vi "Check Buffer Size (Base 2).vi"(5 "source vi name":string, 6 "bytes to move":u64 format="%d bytes", 7 "power of 2":i16, 8 "error in (no error)":errorcluster, 9 "offset (0)":u64 format="%d bytes", 10 "buffer count":u64 format="%d elements", 11 "Pointer in":refnum<class "Pointer.lvclass">) -> (0 "error out":errorcluster, 1 "offset":u64 format="%d bytes", 2 "buffer count":u64 format="%d elements", 3 "Pointer out":refnum<class "Pointer.lvclass">)   [LabVIEW 2017, in "Memory Manager.lvlib" / "Pointer.lvclass"]
uses:
  Pointer.lvclass
  Buffer Underflow.vi
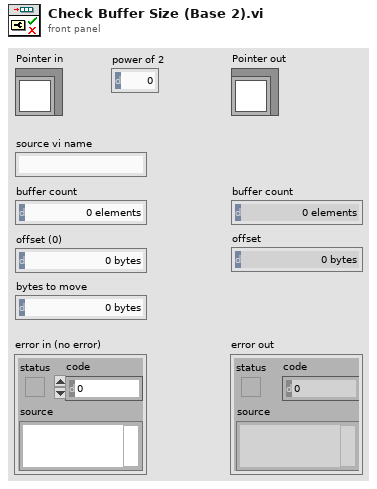
[diagram p1: front panel]
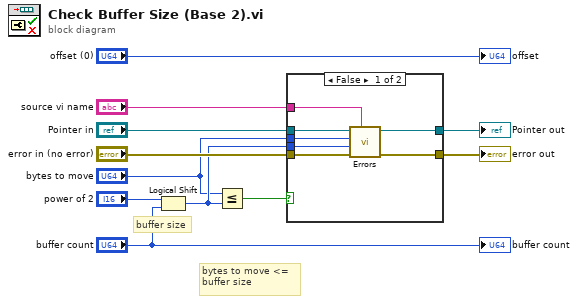
[diagram p0: block diagram]
diagram:
  # "bytes to move <= buffer size"
  # "buffer size"
  n1 = Logical Shift(y="power of 2", x="buffer count") -> (x << y=w4:u64)
  n2 = Less Or Equal?(x="bytes to move", y=w4) -> (x <= y?=w2:bool)
  n3 = case shown="False" w2 {
    tunnel: "Pointer in" -> [w18 w20]
    tunnel: "error in (no error)" -> [w17 w19]
    tunnel: [w16 w19] -> w8
    tunnel: [w15 w20] -> w7
    tunnel: "source vi name" -> [w14 _]
    tunnel: w4 -> [w13 _]
    tunnel: "bytes to move" -> [w12 _]
    frame False {
      n4 = call-poly "Errors.vi"("error source vi name"=w14, "error in (no error)"=w17, "actual buffer size"=w13, "required buffer size"=w12, "Pointer in"=w18) -> ("error out"=w16:errorcluster, "Pointer out"=w15:refnum<class "Pointer.lvclass">)  [unwired: 5 in]
    }
    frame True {
    }
  }
  "error out" <- w8
  "Pointer out" <- w7
  "buffer count" <- "buffer count"
  "offset" <- "offset (0)"
